vi "MGCC_MdlMgmt_RTDS.vi"   [LabVIEW 2016]
uses:
  <vilib>/Utility/error.llb/Error Cluster From Error Code.vi
  <vilib>/ErrorRing/Error Ring.xnode
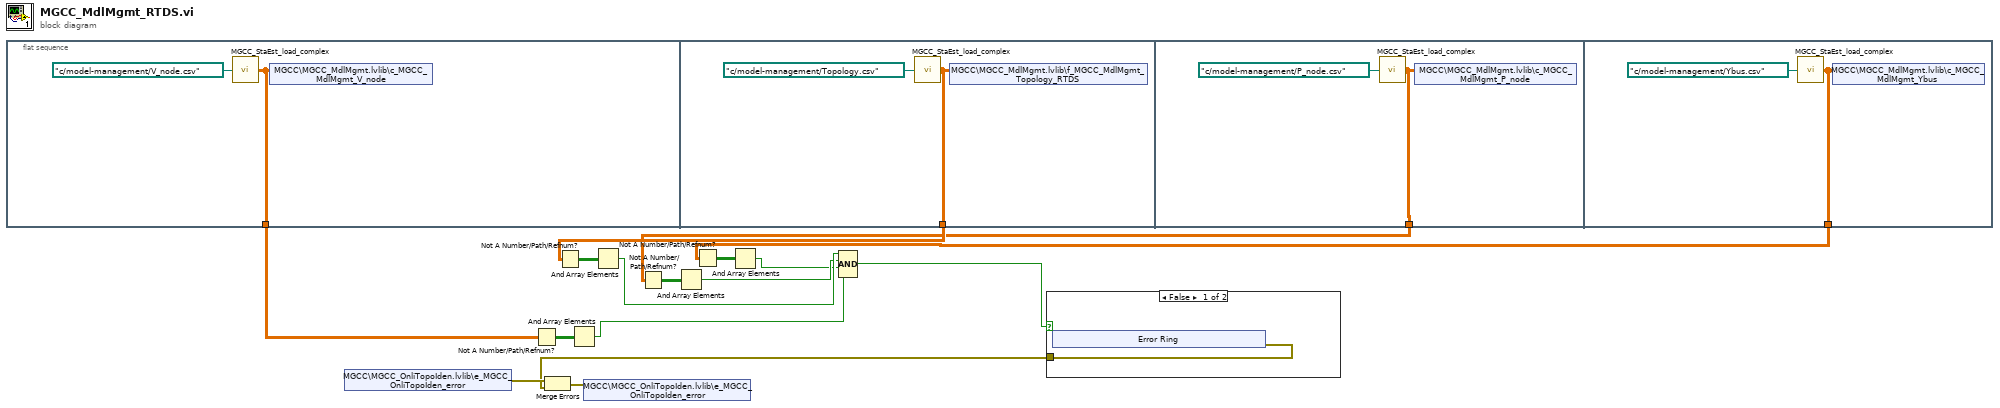
[diagram p0: block diagram]
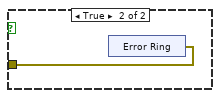
[diagram p2: hidden frame]
diagram:
  n1 = flat-sequence {
    tunnel: [w17] -> w12
    tunnel: [w19] -> w8
    tunnel: [w21] -> w7
    tunnel: [w23] -> w6
    frame #0 {
      n2 = call "MGCC_StaEst_load_complex.vi"("file path (dialog if empty)"=path "c:/model-management/V_node.csv" ("file path (use dialog)")) -> ("Array 13"=w17:cdb[][])
      n3 = shared-variable "MGCC\\MGCC_MdlMgmt.lvlib\\c_MGCC_MdlMgmt_V_node"(w17) -> ()  [unwired: 1 in, 1 out]
    }
    frame #1 {
      n4 = call "MGCC_StaEst_load_complex.vi"("file path (dialog if empty)"=path "c:/model-management/Topology.csv" ("file path (use dialog)")) -> ("Array 13"=w19:cdb[][])
      n5 = shared-variable "MGCC\\MGCC_MdlMgmt.lvlib\\f_MGCC_MdlMgmt_Topology_RTDS"(w19) -> ()  [unwired: 1 in, 1 out]
    }
    frame #2 {
      n6 = call "MGCC_StaEst_load_complex.vi"("file path (dialog if empty)"=path "c:/model-management/P_node.csv" ("file path (use dialog)")) -> ("Array 13"=w21:cdb[][])
      n7 = shared-variable "MGCC\\MGCC_MdlMgmt.lvlib\\c_MGCC_MdlMgmt_P_node"(w21) -> ()  [unwired: 1 in, 1 out]
    }
    frame #3 {
      n8 = call "MGCC_StaEst_load_complex.vi"("file path (dialog if empty)"=path "c:/model-management/Ybus.csv" ("file path (use dialog)")) -> ("Array 13"=w23:cdb[][])
      n9 = shared-variable "MGCC\\MGCC_MdlMgmt.lvlib\\c_MGCC_MdlMgmt_Ybus"(w23) -> ()  [unwired: 1 in, 1 out]
    }
  }
  n10 = shared-variable "MGCC\\MGCC_OnliTopoIden.lvlib\\e_MGCC_OnliTopoIden_error"() -> (w16:errorcluster)  [unwired: 1 in, 1 out]
  n11 = Not A Number/Path/Refnum?(number/path/refnum=w12) -> (NaN/Path/Refnum?=w13:bool[][])
  n12 = Not A Number/Path/Refnum?(number/path/refnum=w8) -> (NaN/Path/Refnum?=w11:bool[][])
  n13 = And Array Elements(Boolean array=w13) -> (logical AND=w2:bool)
  n14 = And Array Elements(Boolean array=w11) -> (logical AND=w5:bool)
  n15 = Not A Number/Path/Refnum?(number/path/refnum=w7) -> (NaN/Path/Refnum?=w9:bool[][])
  n16 = And Array Elements(Boolean array=w9) -> (logical AND=w4:bool)
  n17 = Not A Number/Path/Refnum?(number/path/refnum=w6) -> (NaN/Path/Refnum?=w10:bool[][])
  n18 = And Array Elements(Boolean array=w10) -> (logical AND=w3:bool)
  n19 = Compound Arithmetic op=AND(w5, w4, w3, w2) -> (w1:bool)
  n20 = case shown="False" w1 {
    tunnel: [w25 w31] -> w14
    frame False {
      n21 = xnode "Error Ring"() -> ("error out"=w25:errorcluster)
    }
    frame True {
      n22 = xnode "Error Ring"() -> ("error out"=w31:errorcluster)
    }
  }
  n23 = Merge Errors(w16, w14) -> (w15:errorcluster)
  n24 = shared-variable "MGCC\\MGCC_OnliTopoIden.lvlib\\e_MGCC_OnliTopoIden_error"(w15) -> ()  [unwired: 1 in, 1 out]
